vi "initialize.vi"(8 "error in":errorcluster, 10 "Target Configuration":refnum<class "PL_Target Configuration.lvclass">, 11 "Target Runtime in":refnum<class "PL_Target Runtime.lvclass">) -> (0 "error out":errorcluster, 3 "Target Runtime out":refnum<class "PL_Target Runtime.lvclass">)   [LabVIEW 2013, in "PL_Target Runtime.lvclass"]
doc: "Initializes a target runtime object with a target configuration. This includes initializing target-wide behavior (like loading a bitfile) and caching any associated information or references. Only one target should be initialized per LabVIEW context, and generally only one should be used per hardware device."
uses:
  PL_Target Runtime.lvclass
  target configuration/PL_Target Configuration.lvclass
  target configuration/PL_Target Configuration.lvclass/PL_Target Configuration.ctl
  <vilib>/NI/Tag Bus Module Framework/FPGA manager/methods.ctl
  PL_Target Runtime.lvclass/PL_Target Runtime.ctl
  target configuration/Read load bitfile.vi
  target configuration/Read RIO FPGA.vi
  target configuration/Read bitfile path.vi
  <vilib>/NI/Tag Bus Module Framework/FPGA manager/FPGA manager.lvlib
  <vilib>/NI/Configuration Framework/NISE_CEF_TreeControl.lvlib
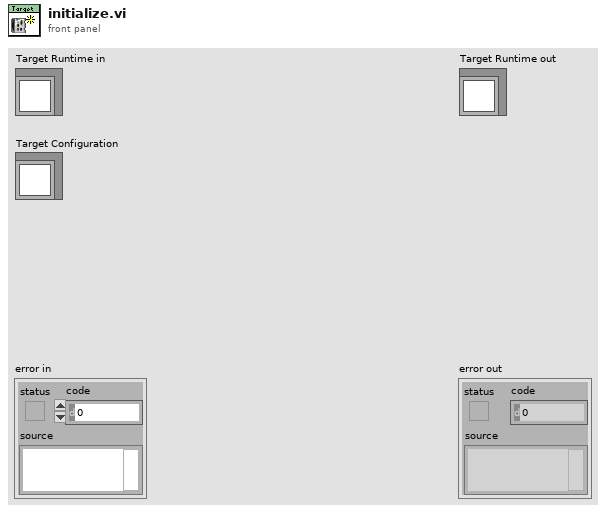
[diagram p1: front panel]
types:
  T1 = typedef "FPGA manager.lvlib/methods.ctl" = enum16{"initialize bitfile", "cache bitfile", "locate bitfile", "close bitfile"}
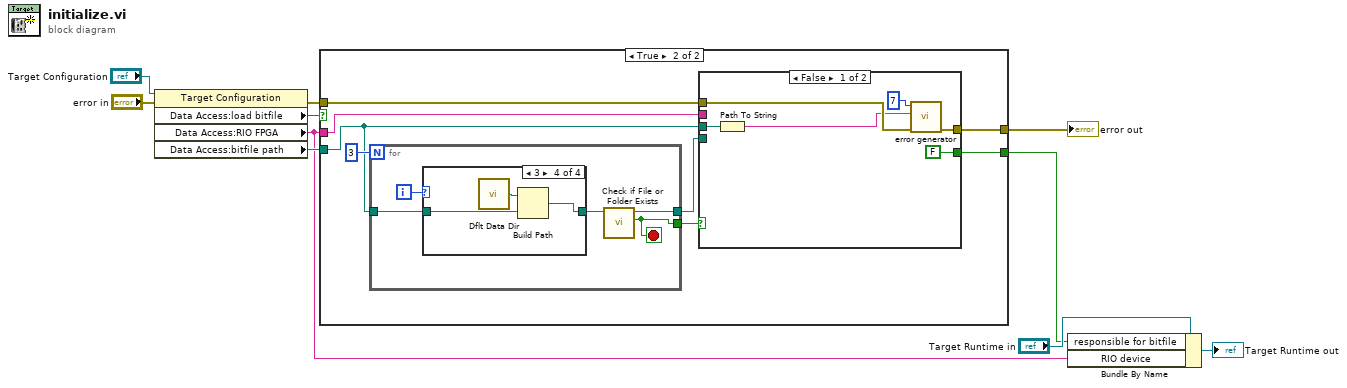
[diagram p0: block diagram]
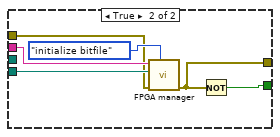
[diagram p3: hidden frame]
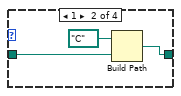
[diagram p5: hidden frame]
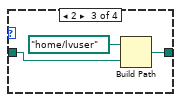
[diagram p6: hidden frame]
diagram:
  n1 = property class="Target Configuration"(reference="Target Configuration", error in="error in") -> (error out=w7:errorcluster, "Data Access:load bitfile"=w4:bool, "Data Access:RIO FPGA"=w1:string, "Data Access:bitfile path"=w6:path)  [unwired: 1 out]
  n2 = case shown="True" w4 {
    selector: w4 -> [w11 _]
    tunnel: w7 -> [w12 w15]
    tunnel: w1 -> [_ w20]
    tunnel: w6 -> [_ w13]
    tunnel: [w12 w19] -> w5
    tunnel: [w11 w18] -> w2
    frame False {
    }
    frame True {
      n3 = for {
        N: 3 -> [_]
        tunnel: w13 -> [w33]
        tunnel: [w36] -> w14
        tunnel: [w35] -> w16
        i -> [w37]
        stop <- w36 stop-if-true
        n4 = case shown="3" w37 {
          tunnel: [w38 w39 w42 w46] -> w34
          tunnel: w33 -> [w38 w40 w43 w47]
          frame ..0, Default {
          }
          frame 1 {
            n5 = Build Path(base path=path "C:/" ("Data Access:bitfile path"), name or relative path=w40) -> (appended path=w39:path)
          }
          frame 2 {
            n6 = Build Path(base path=path "home/lvuser" ("Data Access:bitfile path"), name or relative path=w43) -> (appended path=w42:path)
          }
          frame 3 {
            n7 = call <vilib>:"Dflt Data Dir.vi"() -> ("App:Default Data Directory"=w45:path)
            n8 = Build Path(base path=w45, name or relative path=w47) -> (appended path=w46:path)
          }
        }
        n9 = call <vilib>:"Check if File or Folder Exists.vi"("path"=w34) -> ("file or folder exists?"=w36:bool, "dup path"=w35:path)  [unwired: 8 in, 1 out]
      }
      n10 = case shown="False" w14 {
        tunnel: w20 -> [_ w32]
        tunnel: [w24 w30] -> w19
        tunnel: [FALSE w29] -> w18
        tunnel: w16 -> [_ w28]
        tunnel: w15 -> [w25 w27]
        tunnel: w13 -> [w22 _]
        frame False {
          n11 = Path To String(path=w22) -> (string=w21:string)
          n12 = call <vilib>:"error generator.vi"("error in"=w25, "append error message"=w21, "error code (0)"=7) -> ("error out"=w24:errorcluster)  [unwired: 6 in]
        }
        frame True {
          n13 = call <vilib>:"FPGA manager.vi"("action"=methods."initialize bitfile", "error in"=w27, "Bitfile path"=w28, "RIO resource"=w32) -> ("error out"=w30:errorcluster)  [unwired: 5 in, 2 out]
          n14 = Not(x=w30) -> (.not. x?=w29:bool)
        }
      }
    }
  }
  "error out" <- w5
  n15 = Bundle By Name(cluster="Target Runtime in", "responsible for bitfile"=w2, "RIO device"=w1) -> (→"Target Runtime out":refnum<class "PL_Target Runtime.lvclass">)
